vi "GUI Build PS Vector.vi"(11 "PS Indexes in":i32[](array[numeric])) -> (3 "PS Indexes out":i32[](array[numeric]))   [LabVIEW 2011, in "User Interface VIs.lvlib"]
uses:
  User Interface VIs.lvlib
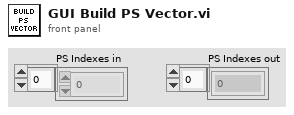
[diagram p1: front panel]
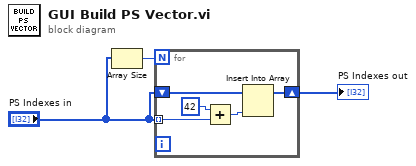
[diagram p0: block diagram]
diagram:
  n1 = Array Size(array="PS Indexes in") -> (size(s)=w1:i32)
  n2 = for {
    N: w1 -> [_]
    shift-right: [w7] -> w3
    shift-left: "PS Indexes in" -> [w8]
    tunnel: "PS Indexes in" -> [w4] mode=indexing
    n3 = Add(x=42, y=w4) -> (x+y=w5:i32)
    n4 = Insert Into Array(array=w8, new element=w5) -> (w7:i32[])  [unwired: 1 in]
  }
  "PS Indexes out" <- w3
